vi "ECC_v4_temp.vi"() -> ()   [LabVIEW 2013]
uses:
  state_machine.ctl
  <vilib>/DAQmx/write.llb/DAQmx Write (Analog Wfm 1Chan NSamp).vi
  <vilib>/DAQmx/create/channels.llb/DAQmx Create Channel (AO-Voltage-Basic).vi
  <vilib>/DAQmx/configure/timing.llb/DAQmx Timing (Use Waveform).vi
  <vilib>/DAQmx/miscellaneous.llb/DAQmx Fill In Error Info.vi
panel:
  in  "temp_rf_on_delay, s":u32
  in  "temp_amp_on_delay, s":u32
  out "AMP_status":bool
  in  "APS/APM":bool=TRUE
  in  "AMP address":tag="Dev1/port0/line0"
  in  "R&S/5181":bool=TRUE
  out "Pause, s":i32
  out "APS_off_status":bool=TRUE
  out "R&S_off_status":bool=TRUE
  out "Countdown":u32
  in  "Rep_delay":u32
  in  "Finite/Continuous":bool
  in  "ResumeSweep":bool
  in  "PauseSweep":bool
  in  "RF_off_rep":bool=TRUE
  in  "RF_off_set":bool
  in  "RF_off_cycle":bool
  in  "APS_off_rep":bool=TRUE
  in  "APS_off_set":bool
  in  "APS_off_cycle":bool
  in  "AbortSweep":bool
  in  "Check APS":bool
  in  "ON/OFF_APS":bool
  in  "Check R&S":bool
  in  "ON/OFF_RF":bool
  in  "Use_APS":bool=TRUE
  out "DAC_status":bool
  out "RF_status":bool
  out "i_Current_repetition":i32
  out "N_Cycles_Created":i32
  out "i_Current_cycle":i32
  in  "M_repetitions":i32 min=0
  in  "Set_of_Cycles":T1(array[cluster])=[{"On/Off"=TRUE, "f0, MHz"=32.5, "fm, kHz"=100, "A, mV"=20, "Waveform"=enum."triangle", "N_steps"=500, "T_sweep, s"=0.1, "N_sweeps"=5, "End_Wait, s"=0}] {"End_Wait, s" step=1; "N_sweeps" min=0 step=1; "T_sweep, s" min=0.0 step=0.001 format="%#_6f"; "N_steps" min=0 step=1; "fm, kHz" step=1; "f0, MHz" min=0.0 step=0.001 format="%#_6f"}
  out "APS_status":bool
  in  "APS address":refnum<visa-resource-name>="COM3"
  in  "Init Devices":bool
  in  "Do Sweep":bool
  in  "Exit":bool
  in  "DAC channel":tag="Dev1/ao0"
  in  "RF address":string(combo)="19"
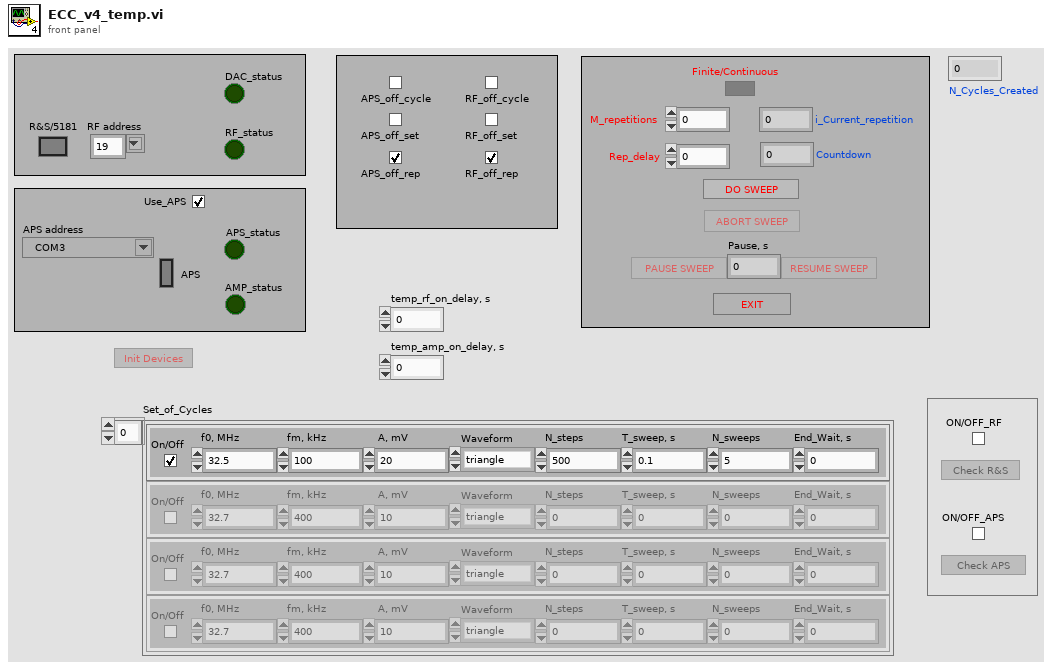
[diagram p1: front panel]
types:
  T1 = cluster{"On/Off":bool, "f0, MHz":dbl, "fm, kHz":i32, "A, mV":i32, "Waveform":enum16{"triangle", "saw_direct", "saw_invert", "sine"}, "N_steps":i32, "T_sweep, s":dbl, "N_sweeps":i32, "End_Wait, s":u32}[]
  T2 = typedef "state_machine.ctl" = enum16{"idle", "init_daq", "init_rf", "init_ps", "cycle_start", "get_wf", "rf_on", "rf_off", "rf_set", "ps_on", "ps_off", "daq_start", "daq_stop", "daq_wait", "daq_dt", "daq_v", "delay", "cycle_reset", "exit", "repetition_reset"}
  T3 = enum8{"Enabled", "Disabled", "Disabled and Grayed Out"}
  T4 = cluster{"On/Off":bool, "f0, MHz":dbl, "fm, kHz":i32, "A, mV":i32, "Waveform":enum16{"triangle", "saw_direct", "saw_invert", "sine"}, "N_steps":i32, "T_sweep, s":dbl, "N_sweeps":i32, "End_Wait, s":u32}
  T5 = enum16{"triangle", "saw_direct", "saw_invert", "sine"}
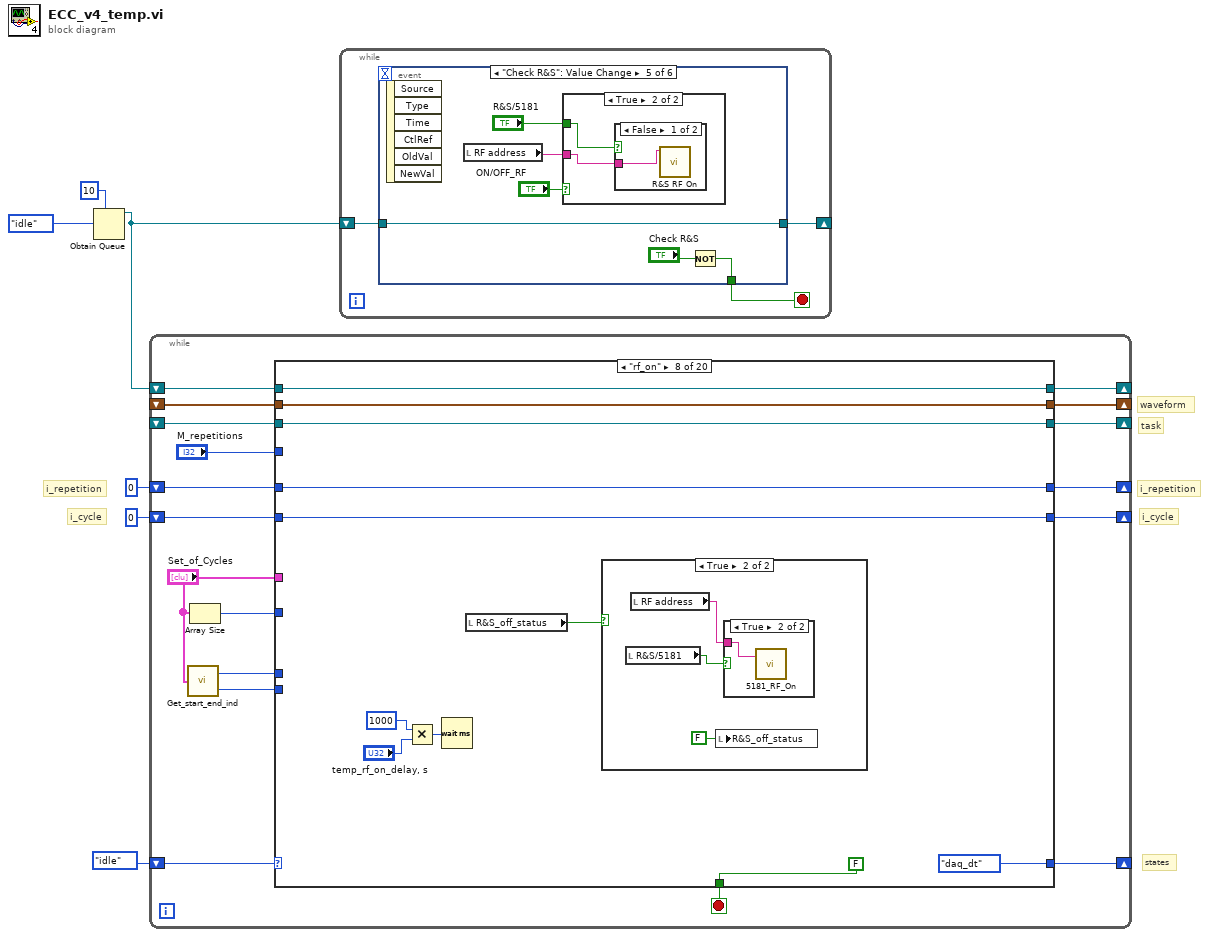
[diagram p0: block diagram]
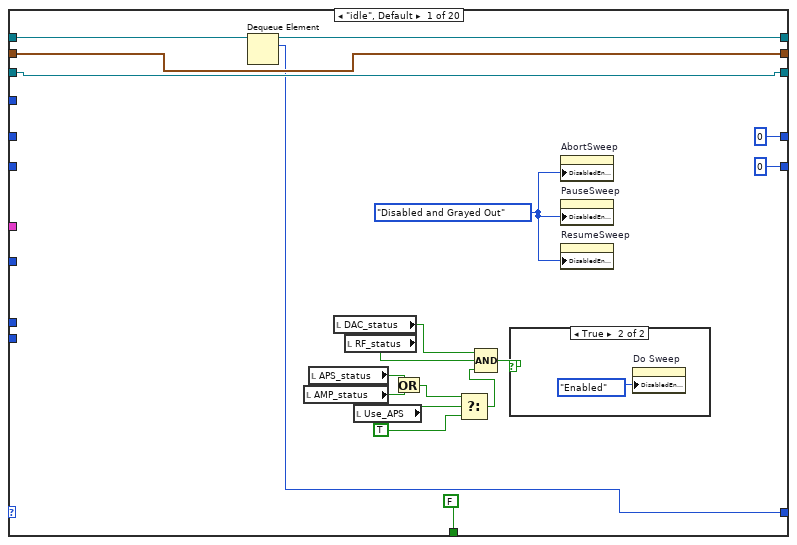
[diagram p2: hidden frame]
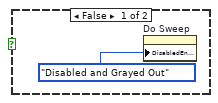
[diagram p3: hidden frame]
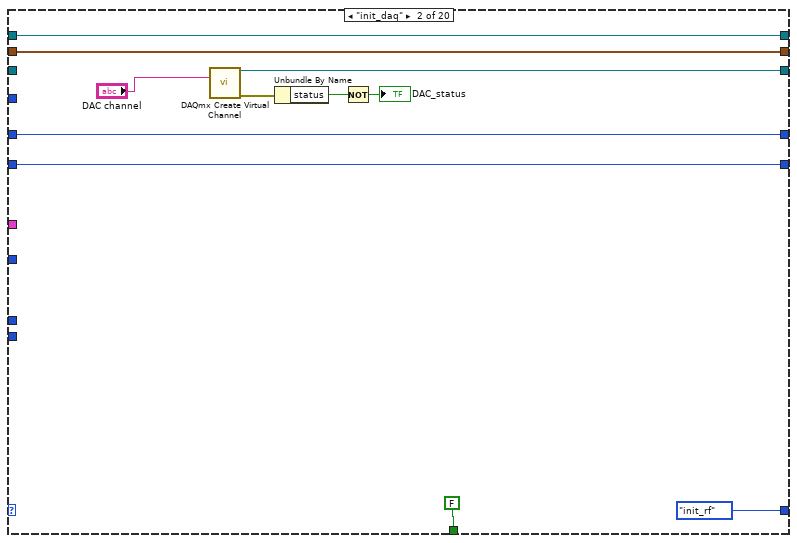
[diagram p4: hidden frame]
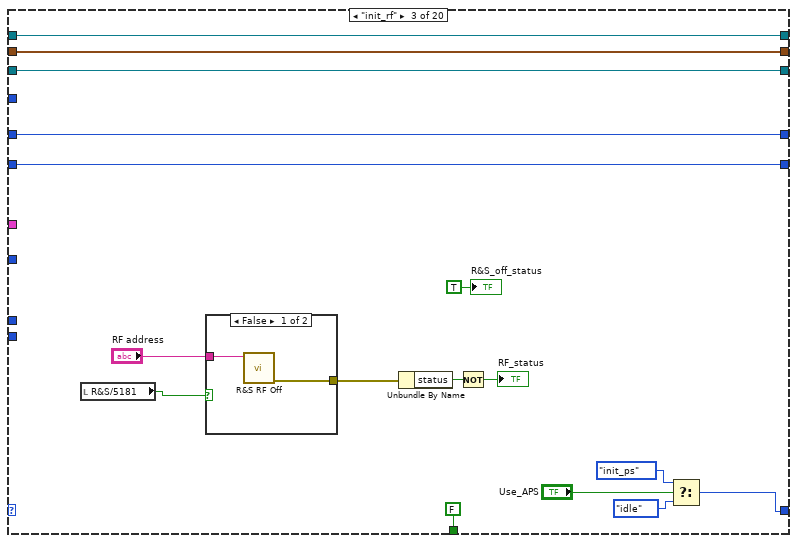
[diagram p5: hidden frame]
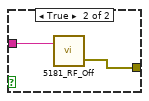
[diagram p6: hidden frame]
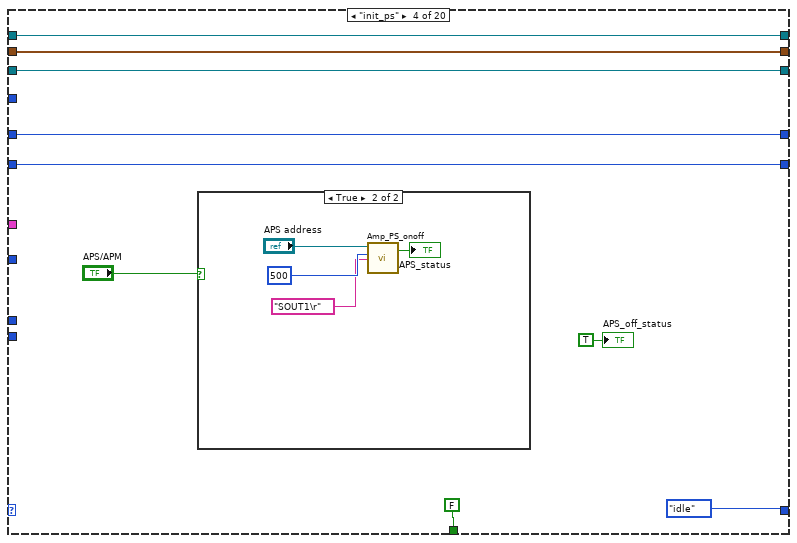
[diagram p7: hidden frame]
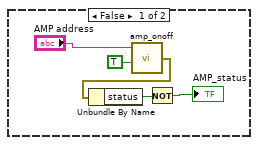
[diagram p8: hidden frame]
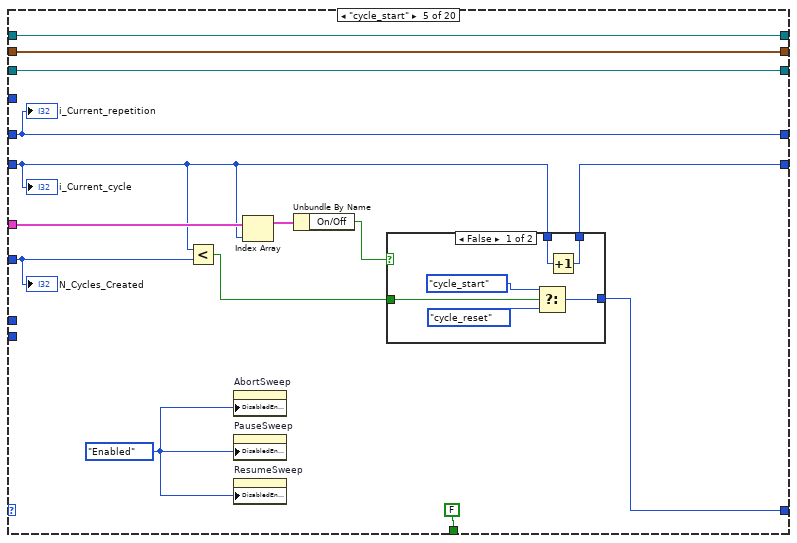
[diagram p9: hidden frame]
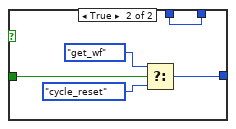
[diagram p10: hidden frame]
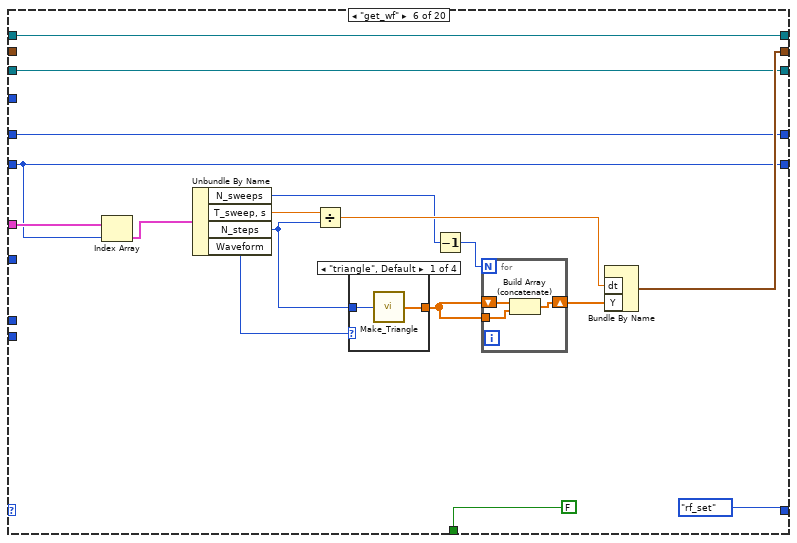
[diagram p11: hidden frame]
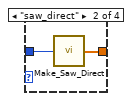
[diagram p12: hidden frame]
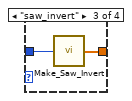
[diagram p13: hidden frame]
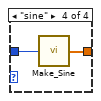
[diagram p14: hidden frame]
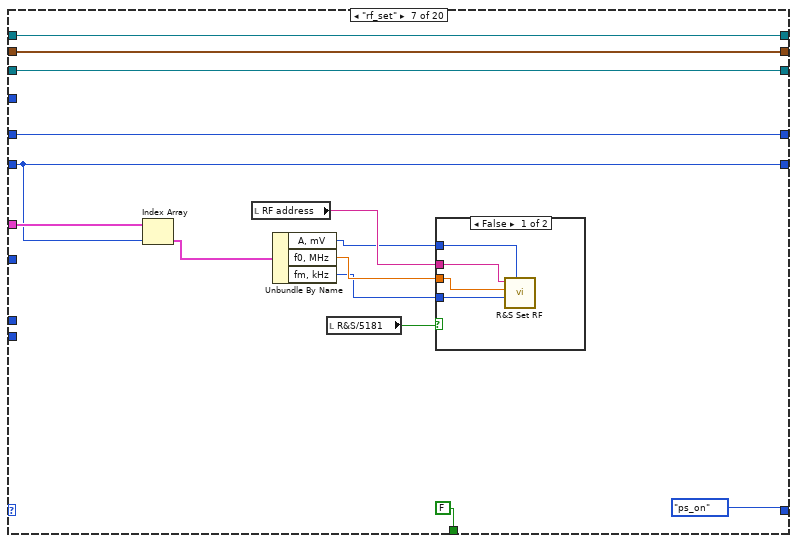
[diagram p15: hidden frame]
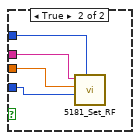
[diagram p16: hidden frame]
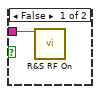
[diagram p18: hidden frame]
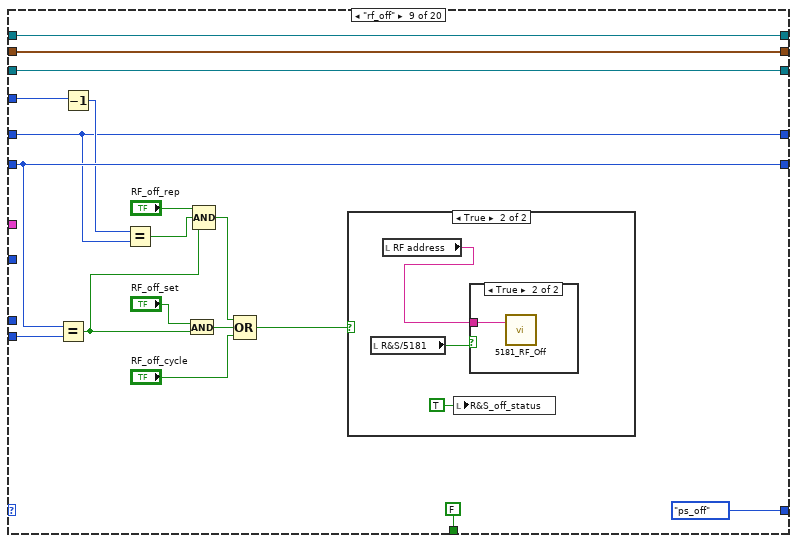
[diagram p19: hidden frame]
diagram:
  # "i_repetition"
  # "i_cycle"
  # "i_repetition"
  # "i_cycle"
  # "states"
  # "waveform"
  # "task"
  n1 = Obtain Queue(max queue size (-1, unlimited)=10, element data type=state_machine."idle") -> (queue out=w4:refnum<queue>)  [unwired: 3 in, 2 out]
  n2 = while {
    shift-right: [w19] -> _
    shift-left: state_machine."idle" -> [w24]
    shift-right: [w23] -> _
    shift-left: _ -> [w21]
    shift-right: [w22] -> _
    shift-left: _ -> [w20]
    shift-right: [w17] -> _
    shift-left: w4 -> [w18]
    shift-right: [w15] -> _
    shift-left: 0 -> [w14]
    shift-right: [w13] -> _
    shift-left: 0 -> [w12]
    stop <- w16 stop-if-true
    n3 = call "Get_start_end_ind.vi"("Set_of_Cycles"="Set_of_Cycles") -> ("start_ind"=w9:i32, "end_ind"=w8:i32)
    n4 = Array Size(array="Set_of_Cycles") -> (size(s)=w11:i32)
    n5 = case shown="\"rf_on\"" w24 {
      selector: w24 -> [_ _ _ _ _ _ _ _ _ _ _ _ _ _ _ _ _ _ w382 _]
      tunnel: [w42 w54 w71 w84 w97 w128 w157 w177 w200 w222 w243 w270 w278 w286 w295 w302 w314 w332 w379 w390] -> w23
      tunnel: "Set_of_Cycles" -> [_ _ _ _ w107 w135 w159 _ _ _ _ _ _ _ _ _ w311 _ _ _]
      tunnel: [w41 w53 w70 w83 w98 w129 w156 w178 w201 w221 w242 w269 w277 w285 w294 w303 w315 w331 w378 w391] -> w22
      tunnel: w21 -> [w42 _ w71 w84 w97 w128 w157 w177 w200 w222 w243 w271 w279 w287 w296 w304 w314 w332 w379 w390]
      tunnel: w20 -> [w41 w53 w70 w83 w98 _ w156 w178 w201 w221 w242 w269 w277 w285 w294 w303 w315 w331 w378 w391]
      tunnel: [w38 state_machine."init_rf" w61 state_machine."idle" w103 state_machine."rf_set" state_machine."ps_on" state_machine."daq_dt" state_machine."ps_off" state_machine."rf_on" state_machine."delay" state_machine."daq_wait" state_machine."rf_off" state_machine."daq_stop" state_machine."daq_v" state_machine."daq_start" state_machine."cycle_start" w330 w382 w386] -> w19
      tunnel: w18 -> [w40 w50 w68 w80 w96 w126 w154 w179 w202 w218 w239 w266 w274 w282 w290 w299 w316 w333 w381 w393]
      tunnel: [w39 w50 w68 w80 w96 w126 w154 w179 w202 w218 w239 w266 w274 w282 w290 w299 w316 w333 w381 w393] -> w17
      tunnel: [FALSE FALSE FALSE FALSE FALSE FALSE FALSE FALSE FALSE FALSE FALSE FALSE FALSE FALSE FALSE FALSE FALSE FALSE TRUE FALSE] -> w16
      tunnel: w11 -> [_ _ _ _ w99 _ _ _ _ _ _ _ _ _ _ _ _ _ _ _]
      tunnel: [0 w49 w67 w79 w102 w119 w152 w173 w196 w216 w237 w265 w273 w281 w289 w298 w306 0 w377 w392] -> w15
      tunnel: w14 -> [_ w49 w67 w79 w100 w119 w152 w173 w196 w216 w237 w265 w273 w281 w289 w298 w305 _ w377 w392]
      tunnel: [0 w48 w66 w78 w95 w121 w153 w176 w188 w217 w233 w264 w272 w280 w288 w297 w313 w327 w376 0] -> w13
      tunnel: w12 -> [_ w48 w66 w78 w95 w121 w153 w176 w188 w217 w233 w264 w272 w280 w288 w297 w313 w328 w376 _]
      tunnel: "M_repetitions" -> [_ _ _ _ _ _ _ _ w193 _ w235 _ _ _ _ _ _ w335 _ _]
      tunnel: w9 -> [_ _ _ _ _ _ _ _ _ _ _ _ _ _ _ _ _ _ _ _]
      tunnel: w8 -> [_ _ _ _ _ _ _ _ w197 _ w238 _ _ _ _ _ _ _ _ _]
      frame "idle", Default {
        w28 = T3."Disabled and Grayed Out" ("Disabled")
        n6 = Dequeue Element(queue=w40) -> (queue out=w39:refnum<queue>, element=w38:T2)  [unwired: 2 in, 2 out]
        n7 = local read "AMP_status"() -> (w26:bool)
        n8 = local read "APS_status"() -> (w27:bool)
        n9 = local read "DAC_status"() -> (w34:bool)
        n10 = local read "RF_status"() -> (w33:bool)
        n11 = local read "Use_APS"() -> (w32:bool)
        n12 = Or(x=w27, y=w26) -> (x .or. y?=w25:bool)
        n13 = Select(t=w25, s=w32, f=TRUE) -> (s? t:f=w30:bool)
        n14 = Compound Arithmetic op=AND(w34, w33, w30) -> (w29:bool)
        n15 = case shown="True" w29 {
          frame False {
            n16 = property on="Do Sweep" class="Bool"("DisabledEnum"=T3."Disabled and Grayed Out" ("Disabled")) -> ()  [unwired: 2 in, 2 out]
          }
          frame True {
            n17 = property on="Do Sweep" class="Bool"("DisabledEnum"=T3."Enabled" ("Disabled")) -> ()  [unwired: 2 in, 2 out]
          }
        }
        n18 = property on="AbortSweep" class="Bool"("DisabledEnum"=w28) -> ()  [unwired: 2 in, 2 out]
        n19 = property on="PauseSweep" class="Bool"("DisabledEnum"=w28) -> ()  [unwired: 2 in, 2 out]
        n20 = property on="ResumeSweep" class="Bool"("DisabledEnum"=w28) -> ()  [unwired: 2 in, 2 out]
      }
      frame "init_daq" {
        n21 = call-poly <vilib>:"DAQmx Create Virtual Channel.vi"("physical channels"="DAC channel") -> ("task out"=w54:refnum<k21>, "error out"=w47:errorcluster)  [unwired: 13 in]
        n22 = Unbundle By Name(w47) -> ("status"=w46:bool)
        n23 = Not(x=w46) -> (.not. x?=→"DAC_status":bool)
      }
      frame "init_rf" {
        n24 = local read "R&S/5181"() -> (w56:bool)
        n25 = case shown="False" w56 {
          tunnel: "RF address" -> [w73 w75]
          tunnel: [w72 w74] -> w57
          frame False {
            n26 = call "R&S RF Off.vi"("address"=w73) -> ("error out"=w72:errorcluster)  [unwired: 5 in, 1 out]
          }
          frame True {
            n27 = call "5181_RF_Off.vi"("address"=w75) -> ("error out"=w74:errorcluster)  [unwired: 1 in, 1 out]
          }
        }
        n28 = Unbundle By Name(w57) -> ("status"=w64:bool)
        n29 = Not(x=w64) -> (.not. x?=→"RF_status":bool)
        n30 = Select(t=state_machine."init_ps", s="Use_APS", f=state_machine."idle") -> (s? t:f=w61:T2)
        "R&S_off_status" <- TRUE ("R&S_off_status")
      }
      frame "init_ps" {
        n31 = case shown="True" "APS/APM" {
          frame False {
            n32 = call "amp_onoff.vi"("amp_onoff"=TRUE, "AMP address"="AMP address") -> ("error out"=w87:errorcluster)  [unwired: 1 in]
            n33 = Unbundle By Name(w87) -> ("status"=w88:bool)
            n34 = Not(x=w88) -> (.not. x?=→"AMP_status":bool)
          }
          frame True {
            n35 = call "Amp_PS_onoff.vi"("On/Off Control"="SOUT1\r", "delay before read (ms)"=u32 500, "Amp PS address"="APS address") -> ("status"=→"APS_status":bool)  [unwired: 1 in, 1 out]
          }
        }
        "APS_off_status" <- TRUE ("APS_off_status")
      }
      frame "cycle_start" {
        w94 = T3."Enabled" ("Disabled")
        n36 = Less?(x=w100, y=w99) -> (x < y?=w104:bool)
        n37 = property on="AbortSweep" class="Bool"("DisabledEnum"=w94) -> ()  [unwired: 2 in, 2 out]
        n38 = property on="PauseSweep" class="Bool"("DisabledEnum"=w94) -> ()  [unwired: 2 in, 2 out]
        n39 = property on="ResumeSweep" class="Bool"("DisabledEnum"=w94) -> ()  [unwired: 2 in, 2 out]
        n40 = Index Array(array=w107, index=w100) -> (element=w106:T4)
        n41 = Unbundle By Name(w106) -> ("On/Off"=w105:bool)
        n42 = case shown="False" w105 {
          tunnel: w104 -> [w111 w117]
          tunnel: [w108 w116] -> w103
          tunnel: w100 -> [w113 w114]
          tunnel: [w112 w114] -> w102
          frame False {
            n43 = Select(t=state_machine."cycle_start", s=w111, f=state_machine."cycle_reset") -> (s? t:f=w108:T2)
            n44 = Increment(x=w113) -> (x+1=w112:i32)
          }
          frame True {
            n45 = Select(t=state_machine."get_wf", s=w117, f=state_machine."cycle_reset") -> (s? t:f=w116:T2)
          }
        }
        "N_Cycles_Created" <- w99
        "i_Current_cycle" <- w100
        "i_Current_repetition" <- w95
      }
      frame "get_wf" {
        n46 = Index Array(array=w135, index=w119) -> (element=w134:T4)
        n47 = Unbundle By Name(w134) -> ("N_sweeps"=w125:i32, "T_sweep, s"=w123:dbl, "N_steps"=w122:i32, "Waveform"=w124:T5)
        n48 = Divide(x=w123, y=w122) -> (x/y=w131:dbl)
        n49 = case shown="\"triangle\", Default" w124 {
          tunnel: w122 -> [w140 w142 w144 w146]
          tunnel: [w139 w141 w143 w145] -> w132
          frame "triangle", Default {
            n50 = call "Make_Triangle.vi"("N_steps_1"=w140) -> ("TriangleWaveform"=w139:dbl[])
          }
          frame "saw_direct" {
            n51 = call "Make_Saw_Direct.vi"("N_steps_1"=w142) -> ("SawDirectWaveform"=w141:dbl[])
          }
          frame "saw_invert" {
            n52 = call "Make_Saw_Invert.vi"("N_steps_1"=w144) -> ("SawInvertWaveform"=w143:dbl[])
          }
          frame "sine" {
            n53 = call "Make_Sine.vi"("N_steps_1"=w146) -> ("SineWaveform"=w145:dbl[])
          }
        }
        n54 = Decrement(x=w125) -> (x-1=w130:i32)
        n55 = for {
          N: w130 -> [_]
          shift-right: [w136] -> w133
          shift-left: w132 -> [w138]
          tunnel: w132 -> [w137]
          n56 = Build Array (concatenate)(w138, w137) -> (w136:dbl[])
        }
        n57 = Bundle By Name("dt"=w131, "Y"=w133) -> (w129:waveform(dbl))  [unwired: 1 in]
      }
      frame "rf_set" {
        n58 = Index Array(array=w159, index=w152) -> (element=w158:T4)
        n59 = local read "RF address"() -> (w160:string)
        n60 = Unbundle By Name(w158) -> ("A, mV"=w151:i32, "f0, MHz"=w150:dbl, "fm, kHz"=w149:i32)
        n61 = local read "R&S/5181"() -> (w147:bool)
        n62 = case shown="False" w147 {
          tunnel: w160 -> [w164 w168]
          tunnel: w151 -> [w163 w167]
          tunnel: w150 -> [w162 w166]
          tunnel: w149 -> [w161 w165]
          frame False {
            n63 = call "R&S Set RF.vi"("amplitude (mV)"=w163, "modulation (kHz)"=w161, "center frequency (MHz)"=w162, "address"=w164) -> ()  [unwired: 3 in, 2 out]
          }
          frame True {
            n64 = call "5181_Set_RF.vi"("address"=w168, "center frequency (MHz)"=w166, "modulation (kHz)"=w165, "amplitude (mV)"=w167) -> ()  [unwired: 1 in, 2 out]
          }
        }
      }
      frame "rf_on" {
        n65 = Multiply(x=u32 1000 ("y"), y="temp_rf_on_delay, s") -> (x*y=w169:u32)
        n66 = Wait (ms)(milliseconds to wait=w169) -> ()  [unwired: 1 out]
        n67 = local read "R&S_off_status"() -> (w172:bool)
        n68 = case shown="True" w172 {
          frame False {
          }
          frame True {
            n69 = local read "R&S/5181"() -> (w180:bool)
            n70 = local read "RF address"() -> (w182:string)
            n71 = local write "R&S_off_status"(FALSE ("R&S_off_status")) -> ()
            n72 = case shown="True" w180 {
              tunnel: w182 -> [w183 w184]
              frame False {
                n73 = call "R&S RF On.vi"("address"=w183) -> ()  [unwired: 5 in, 2 out]
              }
              frame True {
                n74 = call "5181_RF_On.vi"("address"=w184) -> ()  [unwired: 1 in, 2 out]
              }
            }
          }
        }
      }
      frame "rf_off" {
        n75 = Equal?(x=w196, y=w197) -> (x = y?=w185:bool)
        n76 = Decrement(x=w193) -> (x-1=w189:i32)
        n77 = Equal?(x=w189, y=w188) -> (x = y?=w186:bool)
        n78 = And(x="RF_off_set", y=w185) -> (x .and. y?=w192:bool)
        n79 = Compound Arithmetic op=AND("RF_off_rep", w186, w185) -> (w190:bool)
        n80 = Compound Arithmetic op=OR(w190, w192, "RF_off_cycle") -> (w194:bool)
        n81 = case shown="True" w194 {
          frame False {
          }
          frame True {
            n82 = local read "R&S/5181"() -> (w203:bool)
            n83 = local read "RF address"() -> (w205:string)
            n84 = local write "R&S_off_status"(TRUE ("R&S_off_status")) -> ()
            n85 = case shown="True" w203 {
              tunnel: w205 -> [w206 w207]
              frame False {
                n86 = call "R&S RF Off.vi"("address"=w206) -> ()  [unwired: 5 in, 2 out]
              }
              frame True {
                n87 = call "5181_RF_Off.vi"("address"=w207) -> ()  [unwired: 1 in, 2 out]
              }
            }
          }
        }
      }
      frame "ps_on" {
        n88 = local read "APS_status"() -> (w211:bool)
        n89 = local read "APS_status"() -> (w213:bool)
        n90 = Multiply(x=u32 1000 ("y"), y="temp_amp_on_delay, s") -> (x*y=w210:u32)
        n91 = local read "APS_off_status"() -> (w215:bool)
        n92 = Wait (ms)(milliseconds to wait=w210) -> ()  [unwired: 1 out]
        n93 = Or(x=w213, y=w211) -> (x .or. y?=w212:bool)
        n94 = And(x=w212, y=w215) -> (x .and. y?=w214:bool)
        n95 = case shown="True" w214 {
          frame False {
          }
          frame True {
            n96 = local read "APS/APM"() -> (w223:bool)
            n97 = case shown="True" w223 {
              frame False {
                n98 = local read "AMP address"() -> (w225:tag)
                n99 = call "amp_onoff.vi"("amp_onoff"=TRUE, "AMP address"=w225) -> ()  [unwired: 1 in, 1 out]
              }
              frame True {
                n100 = local read "APS address"() -> (w227:refnum<visa-resource-name>)
                n101 = call "Amp_PS_onoff.vi"("On/Off Control"="SOUT0\r", "delay before read (ms)"=u32 500, "Amp PS address"=w227) -> ()  [unwired: 1 in, 2 out]
              }
            }
            n102 = local write "APS_off_status"(FALSE ("APS_off_status")) -> ()
          }
        }
      }
      frame "ps_off" {
        n103 = Decrement(x=w235) -> (x-1=w234:i32)
        n104 = local read "APS_status"() -> (w231:bool)
        n105 = local read "APS_status"() -> (w232:bool)
        n106 = Or(x=w232, y=w231) -> (x .or. y?=w230:bool)
        n107 = case shown="True" w230 {
          selector: w230 -> [w244 _]
          tunnel: w238 -> [_ w256]
          tunnel: w237 -> [_ w255]
          tunnel: [w244 w250] -> w236
          tunnel: w234 -> [_ w246]
          tunnel: w233 -> [_ w247]
          frame False {
          }
          frame True {
            n108 = Equal?(x=w246, y=w247) -> (x = y?=w252:bool)
            n109 = Equal?(x=w255, y=w256) -> (x = y?=w245:bool)
            n110 = Compound Arithmetic op=AND("APS_off_rep", w252, w245) -> (w249:bool)
            n111 = And(x="APS_off_set", y=w245) -> (x .and. y?=w251:bool)
            n112 = Compound Arithmetic op=OR(w249, w251, "APS_off_cycle") -> (w250:bool)
          }
        }
        n113 = case shown="True" w236 {
          frame False {
          }
          frame True {
            n114 = local read "APS/APM"() -> (w257:bool)
            n115 = case shown="True" w257 {
              frame False {
                n116 = local read "AMP address"() -> (w259:tag)
                n117 = call "amp_onoff.vi"("amp_onoff"=FALSE, "AMP address"=w259) -> ()  [unwired: 1 in, 1 out]
              }
              frame True {
                n118 = local read "APS address"() -> (w261:refnum<visa-resource-name>)
                n119 = call "Amp_PS_onoff.vi"("On/Off Control"="SOUT1\r", "delay before read (ms)"=u32 500, "Amp PS address"=w261) -> ()  [unwired: 1 in, 2 out]
              }
            }
            n120 = local write "APS_off_status"(TRUE ("APS_off_status")) -> ()
          }
        }
      }
      frame "daq_start" {
        n121 = call <vilib>:"DAQmx Start Task.vi"("task/channels in"=w271) -> ("task out"=w270:refnum<k21>)  [unwired: 13 in, 1 out]
      }
      frame "daq_stop" {
        n122 = call <vilib>:"DAQmx Stop Task.vi"("task/channels in"=w279) -> ("task out"=w278:refnum<k21>)  [unwired: 13 in, 1 out]
      }
      frame "daq_wait" {
        n123 = call <vilib>:"DAQmx Wait Until Done.vi"("task/channels in"=w287) -> ("task out"=w286:refnum<k21>)  [unwired: 13 in, 1 out]
      }
      frame "daq_dt" {
        w293 = 10178 items=["Finite Samples"=10178, "Continuous Samples"=10123, "Hardware Timed Single Point"=12522] ("sample mode")
        n124 = call-poly <vilib>:"DAQmx Timing.vi"("task/channels in"=w296, "sample mode"=w293, "waveform"=w294) -> ("task out"=w295:refnum<k21>)  [unwired: 11 in, 1 out]
      }
      frame "daq_v" {
        n125 = call-poly <vilib>:"DAQmx Write.vi"("task/channels in"=w304, "data"=w303) -> ("task out"=w302:refnum<k21>)  [unwired: 11 in, 2 out]
      }
      frame "delay" {
        # "iterate cycle"
        n126 = Increment(x=w305) -> (x+1=w306:i32)
        n127 = Index Array(array=w311, index=w305) -> (element=w312:T4)
        n128 = Unbundle By Name(w312) -> ("End_Wait, s"=w309:u32)
        n129 = Equal To 0?(x=w309) -> (x = 0?=w310:bool)
        n130 = case shown="False" w310 {
          tunnel: w309 -> [w317 _]
          frame False {
            n131 = Multiply(x=u32 1000 ("y"), y=w317) -> (x*y=w319:u32)
            n132 = Wait (ms)(milliseconds to wait=w319) -> ()  [unwired: 1 out]
          }
          frame True {
          }
        }
      }
      frame "cycle_reset" {
        # "iterate repetition"
        n133 = Increment(x=w328) -> (x+1=w320:i32)
        n134 = case shown="True" "PauseSweep" {
          selector: "PauseSweep" -> [w347 _]
          tunnel: [w347 w348] -> w324
          frame False {
          }
          frame True {
            n135 = Tick Count (ms)() -> (millisecond timer value=w349:u32)
            n136 = while {
              tunnel: w349 -> [w355]
              tunnel: ["ResumeSweep"] -> w348
              stop <- "ResumeSweep" stop-if-true
              n137 = Tick Count (ms)() -> (millisecond timer value=w356:u32)
              n138 = Subtract(x=w356, y=w355) -> (x-y=w354:u32)
              n139 = Divide(x=w354, y=u32 1000) -> (x/y=w352:dbl)
              n140 = To Long Integer(number=w352) -> (32bit integer=→"Pause, s":i32)
            }
          }
        }
        n141 = Less?(x=w320, y=w335) -> (x < y?=w329:bool)
        n142 = Or(x="AbortSweep", y="PauseSweep") -> (x .or. y?=w321:bool)
        n143 = case shown="False" "AbortSweep" {
          tunnel: [w365 state_machine."idle"] -> w330
          tunnel: w329 -> [w364 _]
          tunnel: w320 -> [w363 _]
          tunnel: [w363 0] -> w327
          frame False {
            n144 = Select(t=state_machine."cycle_start", s=w364, f=state_machine."repetition_reset") -> (s? t:f=w365:T2)
          }
          frame True {
            w369 = T3."Enabled" ("Disabled")
            n145 = property on="Check APS" class="Bool"("DisabledEnum"=w369) -> ()  [unwired: 2 in, 2 out]
            n146 = property on="Check R&S" class="Bool"("DisabledEnum"=w369) -> ()  [unwired: 2 in, 2 out]
          }
        }
        n147 = local read "APS_status"() -> (w322:bool)
        n148 = And(x=w321, y=w322) -> (x .and. y?=w323:bool)
        n149 = case shown="True" w321 {
          frame False {
          }
          frame True {
            n150 = local write "R&S_off_status"(TRUE ("R&S_off_status")) -> ()
            n151 = local read "RF address"() -> (w358:string)
            n152 = call "R&S RF Off.vi"("address"=w358) -> ()  [unwired: 5 in, 2 out]
          }
        }
        n153 = case shown="True" w324 {
          frame False {
          }
          frame True {
            n154 = local read "R&S_off_status"() -> (w342:bool)
            n155 = case shown="False" w342 {
              frame False {
                n156 = local read "RF address"() -> (w346:string)
                n157 = call "R&S RF On.vi"("address"=w346) -> ()  [unwired: 5 in, 2 out]
              }
              frame True {
              }
            }
            n158 = local write "Pause, s"(0 ("Pause, s")) -> ()
            n159 = local read "APS_off_status"() -> (w340:bool)
            n160 = local read "APS_status"() -> (w341:bool)
            n161 = Not(x=w340) -> (.not. x?=w339:bool)
            n162 = And(x=w341, y=w339) -> (x .and. y?=w338:bool)
            n163 = case shown="True" w338 {
              frame False {
              }
              frame True {
                n164 = local read "APS address"() -> (w343:refnum<visa-resource-name>)
                n165 = call "Amp_PS_onoff.vi"("On/Off Control"="SOUT0\r", "delay before read (ms)"=u32 50, "Amp PS address"=w343) -> ()  [unwired: 1 in, 2 out]
              }
            }
          }
        }
        n166 = case shown="True" w323 {
          frame False {
          }
          frame True {
            n167 = local read "APS address"() -> (w360:refnum<visa-resource-name>)
            n168 = local write "APS_off_status"(TRUE ("APS_off_status")) -> ()
            n169 = call "Amp_PS_onoff.vi"("On/Off Control"="SOUT1\r", "delay before read (ms)"=u32 500, "Amp PS address"=w360) -> ()  [unwired: 1 in, 2 out]
          }
        }
      }
      frame "exit" {
        w371 = FALSE ("DAC_status")
        n170 = local read "APS address"() -> (w374:refnum<visa-resource-name>)
        n171 = local read "Use_APS"() -> (w375:bool)
        n172 = local read "RF address"() -> (w373:string)
        n173 = case shown="False" w375 {
          tunnel: w374 -> [_ w383]
          frame False {
          }
          frame True {
            n174 = call "Amp_PS_onoff.vi"("On/Off Control"="SOUT1\r", "delay before read (ms)"=u32 50, "Amp PS address"=w383) -> ()  [unwired: 1 in, 2 out]
          }
        }
        n175 = call "R&S RF Off.vi"("address"=w373) -> ()  [unwired: 5 in, 2 out]
        n176 = property on="Init Devices" class="Bool"("DisabledEnum"=T3."Enabled" ("Disabled")) -> ()  [unwired: 2 in, 2 out]
        n177 = local write "DAC_status"(w371) -> ()
        n178 = local write "RF_status"(w371) -> ()
        n179 = local write "APS_status"(w371) -> ()
      }
      frame "repetition_reset" {
        n180 = case shown="True" "Finite/Continuous" {
          tunnel: [state_machine."idle" state_machine."cycle_start"] -> w386
          frame False {
          }
          frame True {
            n181 = Tick Count (ms)() -> (millisecond timer value=w396:u32)
            n182 = while {
              tunnel: w396 -> [w403]
              tunnel: "Rep_delay" -> [w399]
              stop <- w401 stop-if-true
              w398 = u32 1000 ("y")
              n183 = Tick Count (ms)() -> (millisecond timer value=w404:u32)
              n184 = Subtract(x=w404, y=w403) -> (x-y=w405:u32)
              n185 = Divide(x=w405, y=w398) -> (x/y=w406:dbl)
              n186 = Wait (ms)(milliseconds to wait=w398) -> ()  [unwired: 1 out]
              n187 = To Long Integer(number=w406) -> (32bit integer=w400:i32)
              n188 = Subtract(x=w399, y=w400) -> (x-y=w402:u32)
              "Countdown" <- w402
              n189 = Less Or Equal To 0?(x=w402) -> (x <= 0?=w401:bool)
            }
          }
        }
      }
    }
  }
  n190 = while {
    shift-right: [w407] -> _
    shift-left: w4 -> [w408]
    stop <- w409 stop-if-true
    n191 = event shown="[4] \"Check R&S\": Value Change" {
      selector: _ -> [_ _ _ _ _ _]
      dyn-events: _ -> [_ _ _ _ _ _]
      timeout: _ -> [_ _ _ _ _ _]
      tunnel: [_ "Exit" w419 w425 w432 w445] -> w409
      tunnel: w408 -> [w410 w413 w418 w424 w429 w442]
      tunnel: [w410 w412 w417 w423 w429 w442] -> w407
      event Timeout {
        n192 = event-data() -> ()  [unwired: 1 in, 3 out]
      }
      event "Exit": Value Change {
        n193 = event-data() -> ()  [unwired: 1 in, 6 out]
        n194 = Enqueue Element(queue=w413, element=state_machine."exit") -> (queue out=w412:refnum<queue>)  [unwired: 2 in, 2 out]
      }
      event "Init Devices": Value Change {
        n195 = event-data() -> ()  [unwired: 1 in, 6 out]
        n196 = Enqueue Element(queue=w418, element=state_machine."init_daq") -> (queue out=w417:refnum<queue>)  [unwired: 2 in, 2 out]
        n197 = property on="Init Devices" class="Bool"("DisabledEnum"=T3."Disabled and Grayed Out" ("Disabled")) -> ()  [unwired: 2 in, 2 out]
        n198 = Not(x="Init Devices") -> (.not. x?=w419:bool)
      }
      event "Do Sweep": Value Change {
        w421 = T3."Disabled and Grayed Out" ("Disabled")
        n199 = event-data() -> ()  [unwired: 1 in, 6 out]
        n200 = Enqueue Element(queue=w424, element=state_machine."cycle_start") -> (queue out=w423:refnum<queue>)  [unwired: 2 in, 2 out]
        n201 = Not(x="Do Sweep") -> (.not. x?=w425:bool)
        n202 = property on="Check R&S" class="Bool"("DisabledEnum"=w421) -> ()  [unwired: 2 in, 2 out]
        n203 = property on="Check APS" class="Bool"("DisabledEnum"=w421) -> ()  [unwired: 2 in, 2 out]
      }
      event "Check R&S": Value Change {
        n204 = event-data() -> ()  [unwired: 1 in, 6 out]
        n205 = local read "RF address"() -> (w430:string)
        n206 = case shown="True" "ON/OFF_RF" {
          tunnel: w430 -> [w434 w438]
          tunnel: "R&S/5181" -> [w433 w437]
          frame False {
            n207 = case shown="True" w433 {
              tunnel: w434 -> [w435 w436]
              frame False {
                n208 = call "R&S RF Off.vi"("address"=w435) -> ()  [unwired: 5 in, 2 out]
              }
              frame True {
                n209 = call "5181_RF_Off.vi"("address"=w436) -> ()  [unwired: 1 in, 2 out]
              }
            }
          }
          frame True {
            n210 = case shown="False" w437 {
              tunnel: w438 -> [w439 w440]
              frame False {
                n211 = call "R&S RF On.vi"("address"=w439) -> ()  [unwired: 5 in, 2 out]
              }
              frame True {
                n212 = call "5181_RF_On.vi"("address"=w440) -> ()  [unwired: 1 in, 2 out]
              }
            }
          }
        }
        n213 = Not(x="Check R&S") -> (.not. x?=w432:bool)
      }
      event "Check APS": Value Change {
        n214 = event-data() -> ()  [unwired: 1 in, 6 out]
        n215 = local read "APS address"() -> (w443:refnum<visa-resource-name>)
        n216 = case shown="False" "ON/OFF_APS" {
          tunnel: w443 -> [w446 w449]
          frame False {
            n217 = call "Amp_PS_onoff.vi"("On/Off Control"="SOUT1\r", "delay before read (ms)"=u32 50, "Amp PS address"=w446) -> ()  [unwired: 1 in, 2 out]
          }
          frame True {
            n218 = call "Amp_PS_onoff.vi"("On/Off Control"="SOUT0\r", "delay before read (ms)"=u32 50, "Amp PS address"=w449) -> ()  [unwired: 1 in, 2 out]
          }
        }
        n219 = Not(x="Check APS") -> (.not. x?=w445:bool)
      }
    }
  }
